vi "User Authentication Schemes.vi"(7 "Address":string="localhost", 8 "Error In":errorcluster) -> (0 "Error Out":errorcluster)   [LabVIEW 2017, in "Tests.lvlib" / "Session.lvlib"]
uses:
  Session.lvlib
  src/Toolkit/API/Session/API/Typedefs/User Authentication Schemes.ctl
  <vilib>/addons/_JKI Toolkits/Caraya/classes/Test/Test.lvclass
  src/Toolkit/Toolkit.lvlib
  src/Toolkit/API/Session/Session.lvclass
  <vilib>/addons/_JKI Toolkits/Caraya/classes/Assert/Assert.lvclass
  Tests.lvlib
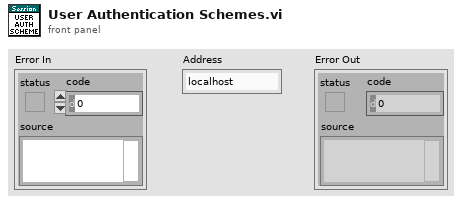
[diagram p1: front panel]
types:
  T1 = typedef "Toolkit.lvlib/Session.lvclass/User Authentication Schemes.ctl" = enum16{"Keyboard", "Password", "Public Key"}
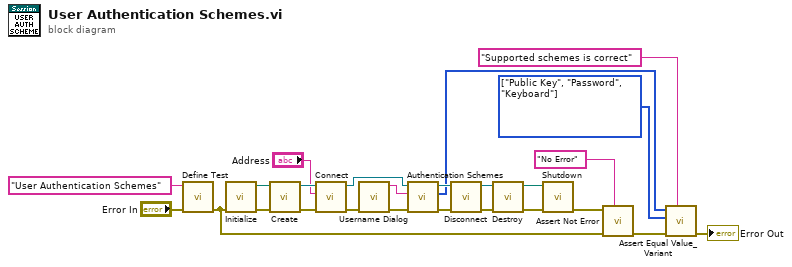
[diagram p0: block diagram]
diagram:
  w4 = T1[] [enum."Public Key", enum."Password", enum."Keyboard"] items=["Keyboard", "Password", "Public Key"] ("Supported Schemes")
  n1 = call <vilib>:"Define Test.vi"("error in (no error)"="Error In", "Label (VI Title)"="User Authentication Schemes") -> ("error out"=w17:errorcluster)  [unwired: 9 in]
  n2 = call "Initialize.vi"("Error In"=w17) -> ("Error Out"=w23:errorcluster, "lv-libssh2 Shared Library Out"=w22:path)  [unwired: 9 in]
  n3 = call "Create.vi"("Error In"=w23, "lv-libssh2 Shared Library"=w22) -> ("Error Out"=w15:errorcluster, "Sesssion"=w16:refnum<class "Session.lvclass">)  [unwired: 8 in]
  n4 = call "Connect.vi"("Error In"=w15, "Address"="Address", "Session In"=w16) -> ("Error Out"=w3:errorcluster, "Sesssion Out"=w11:refnum<class "Session.lvclass">)  [unwired: 7 in]
  n5 = call "Username Dialog.vi"("Error In"=w3) -> ("Error Out"=w2:errorcluster, "Username Out"=w1:string)  [unwired: 9 in]
  n6 = call "Authentication Schemes.vi"("Error In"=w2, "Username"=w1, "Session In"=w11) -> ("Error Out"=w9:errorcluster, "Supported Schemes"=w5:T1[], "Sesssion Out"=w10:refnum<class "Session.lvclass">)  [unwired: 6 in]
  n7 = call "Disconnect.vi"("Error In"=w9, "Session In"=w10) -> ("Error Out"=w12:errorcluster, "Sesssion Out"=w13:refnum<class "Session.lvclass">)  [unwired: 8 in]
  n8 = call "Destroy.vi"("Error In"=w12, "Session"=w13) -> ("Error Out"=w20:errorcluster, "lv-libssh2 Shared Library"=w21:path)  [unwired: 8 in]
  n9 = call "Shutdown.vi"("Error In"=w20, "lv-libssh2 Shared Library"=w21) -> ("Error Out"=w19:errorcluster)  [unwired: 9 in]
  n10 = call <vilib>:"Assert Not Error.vi"("Label"="No Error", "error in (no error)"=w17, "Not Error?"=w19) -> ("error out"=w8:errorcluster)  [unwired: 8 in]
  n11 = call <vilib>:"Assert Equal Value_Variant.vi"("Label"="Supported schemes is correct", "error in (no error)"=w8, "Y"=w4, "X"=w5) -> ("error out"=→"Error Out":errorcluster)  [unwired: 7 in]
